vi "Page_Service_Config_WriteAll.vi"(6 "ctl references":T1, 8 "error in (no error)":errorcluster, 11 "AB_WebService in":refnum<class "AB_WebService.lvclass">) -> (0 "error out":errorcluster, 3 "AB_WebService out":refnum<class "AB_WebService.lvclass">)   [LabVIEW 2020, in "AB_WebService.lvclass"]
uses:
  <vilib>/AppBuilder/AB_Classes/WebService/AB_WebService.lvclass
  <resource>/Framework/Providers/Builds/AppBuilder/AB_UI_Page_Service_Config_References.ctl
  <vilib>/AppBuilder/AB_Classes/WebService/AB_WebService.lvclass/AB_WebService.ctl
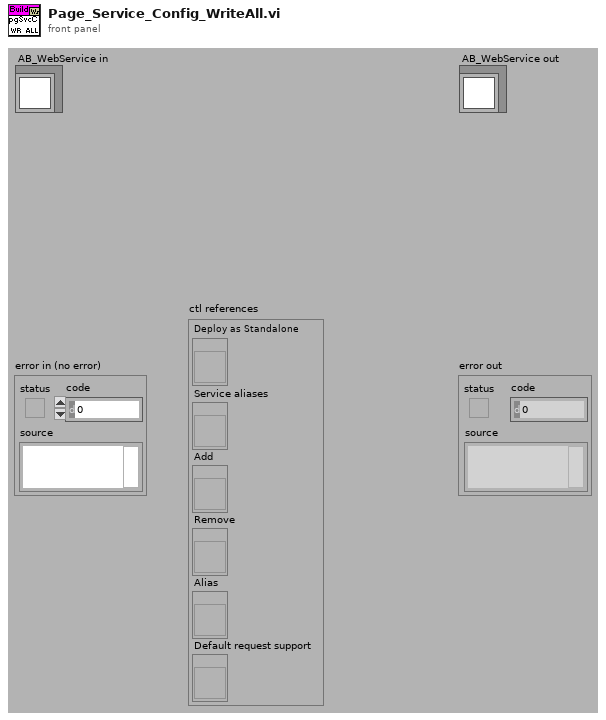
[diagram p1: front panel]
types:
  T1 = typedef "AB_UI_Page_Service_Config_References.ctl" = cluster{"Service aliases":refnum<vi>, "Add":refnum<vi>, "Remove":refnum<vi>, "Alias":refnum<vi>, "Default request support":refnum<vi>, "Deploy as Standalone":refnum<vi>}
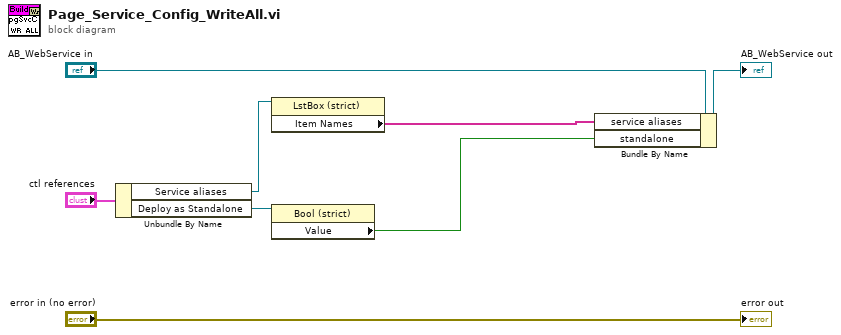
[diagram p0: block diagram]
diagram:
  n1 = Unbundle By Name("ctl references") -> ("Service aliases"=w3:refnum<vi>, "Deploy as Standalone"=w4:refnum<vi>)
  n2 = property class="LstBox (strict)"(reference=w3) -> ("Item Names"=w2:string[])  [unwired: 1 in, 2 out]
  n3 = property class="Bool (strict)"(reference=w4) -> ("Value"=w1:bool)  [unwired: 1 in, 2 out]
  n4 = Bundle By Name(cluster="AB_WebService in", "service aliases"=w2, "standalone"=w1) -> (→"AB_WebService out":refnum<class "AB_WebService.lvclass">)
  "error out" <- "error in (no error)"
